vi "Insert into Subpanel.vi"(8 "error in (no error)":errorcluster, 10 "SubPanel":refnum<vi>, 11 "Missing VI Type in":refnum<class "Missing VI Type.lvclass">) -> (0 "error out":errorcluster, 3 "Missing VI Type out":refnum<class "Missing VI Type.lvclass">)   [LabVIEW 2020, in "Peek Window.lvlib" / "Missing VI Type.lvclass"]
uses:
  Missing VI Type.lvclass
  Missing VI Message.vi
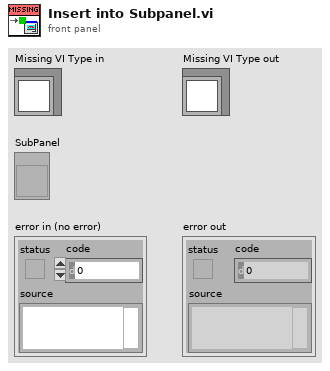
[diagram p1: front panel]
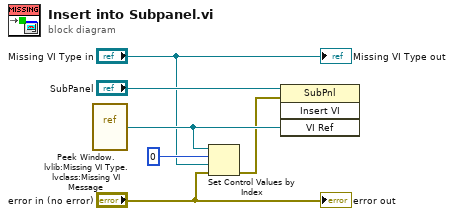
[diagram p0: block diagram]
diagram:
  n1 = vi-ref "Peek Window.lvlib:Missing VI Type.lvclass:Missing VI Message.vi"() -> (w5:refnum<vi>)
  n2 = Set Control Values by Index(0:w5, 1:0, 2:"Missing VI Type in", 3:"error in (no error)") -> (11:w3:errorcluster)
  n3 = invoke class="SubPnl" method="Insert VI"(reference="SubPanel", error in=w3, "VI Ref"=w5) -> ()  [unwired: 1 in, 4 out]
  "error out" <- "error in (no error)"
  "Missing VI Type out" <- "Missing VI Type in"
